vi "ge_GrantCoerceRing.vi"(4 "String and Values":cluster{"String":string, "Value":u16}[](array[cluster]), 5 "Requested Value":u16) -> (2 "Cel Val and Color":cluster{"Value":string, "Color":u32})   [LabVIEW 2012]
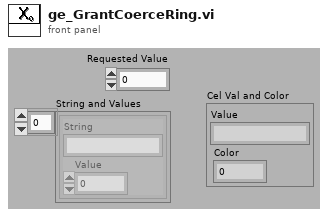
[diagram p1: front panel]
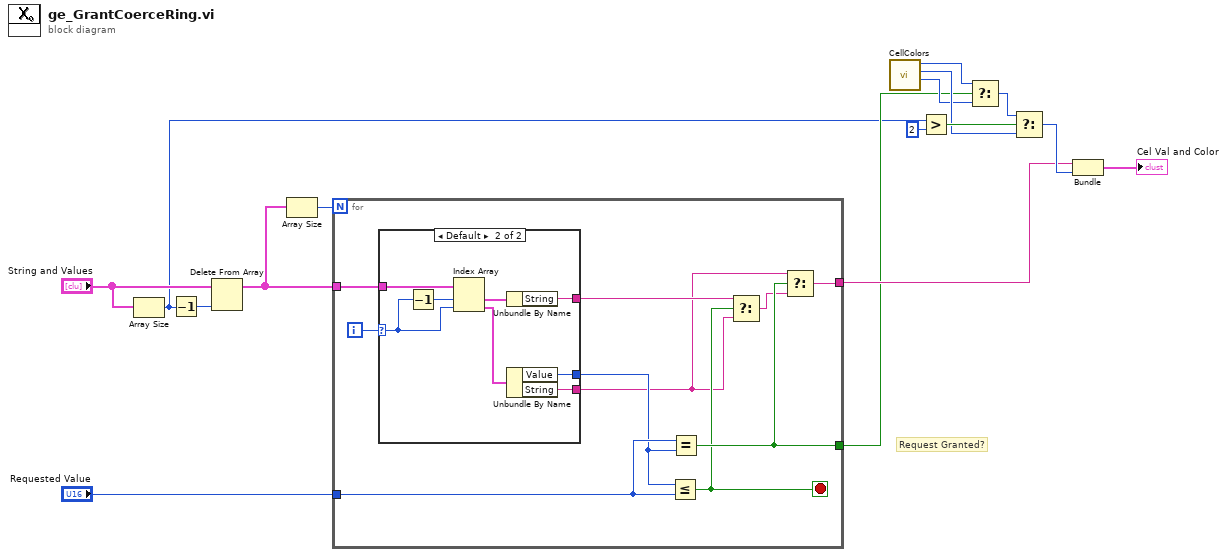
[diagram p0: block diagram]
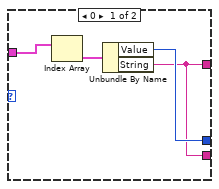
[diagram p2: hidden frame]
diagram:
  # "Request Granted?"
  n1 = Array Size(array="String and Values") -> (size(s)=w3:i32)
  n2 = Decrement(x=w3) -> (x-1=w12:i32)
  n3 = Delete From Array(array="String and Values", index=w12) -> (array with subset deleted=w14:cluster{"String":string, "Value":u16}[])  [unwired: 1 in, 1 out]
  n4 = Array Size(array=w14) -> (size(s)=w16:i32)
  n5 = for {
    N: w16 -> [_]
    tunnel: w14 -> [w26]
    tunnel: "Requested Value" -> [w25]
    tunnel: [w23] -> w4
    tunnel: [w24] -> w5
    i -> [w20]
    stop <- w22 stop-if-true
    n6 = case shown="Default" w20 {
      selector: w20 -> [_ w36]
      tunnel: w26 -> [w30 w38]
      tunnel: [w28 w33] -> w19
      tunnel: [w27 w32] -> w18
      tunnel: [w27 w31] -> w17
      frame 0 {
        n7 = Index Array(array=w30) -> (element=w29:cluster{"String":string, "Value":u16})  [unwired: 1 in]
        n8 = Unbundle By Name(w29) -> ("Value"=w28:u16, "String"=w27:string)
      }
      frame Default {
        n9 = Decrement(x=w36) -> (x-1=w37:i32)
        n10 = Index Array(array=w38, index #1=w37, index #2=w36) -> (element #1=w35:cluster{"String":string, "Value":u16}, element #2=w34:cluster{"String":string, "Value":u16})
        n11 = Unbundle By Name(w35) -> ("String"=w32:string)
        n12 = Unbundle By Name(w34) -> ("Value"=w33:u16, "String"=w31:string)
      }
    }
    n13 = Less Or Equal?(x=w19, y=w25) -> (x <= y?=w22:bool)
    n14 = Equal?(x=w25, y=w19) -> (x = y?=w23:bool)
    n15 = Select(t=w18, s=w22, f=w17) -> (s? t:f=w21:string)
    n16 = Select(t=w17, s=w23, f=w21) -> (s? t:f=w24:string)
  }
  n17 = call "CellColors.vi"() -> ("Coerced"=w7:u32, "Disabled"=w8:u32, "Normal"=w2:u32)  [unwired: 8 in, 1 out]
  n18 = Greater?(x=w3, y=2) -> (0:w9:bool)
  n19 = Select(t=w2, s=w4, f=w7) -> (s? t:f=w10:u32)
  n20 = Select(t=w10, s=w9, f=w8) -> (s? t:f=w6:u32)
  n21 = Bundle("String"=w5, "Disabled"=w6) -> (→"Cel Val and Color":cluster{"String":string, "Disabled":u32})  [unwired: 1 in]
